vi "macro_BoolCmd_RecvMultiplexer.vi"() -> ()   [LabVIEW 2019, in "Trajectory_Library.lvlib"]
uses:
  VI/BoolCmd_Recv_Internal.vi
  VI/DigSeqLogic_Edge_On.vi
  VI/BoolCmd_ObtainQueue.vi
  Trajectory_Library.lvlib
panel:
  in  "Ready2":bool=TRUE
  out "Do Cancel":bool
  out "Do Command 2":bool
  out "Do Command 1":bool
  in  "Ready1":bool=TRUE
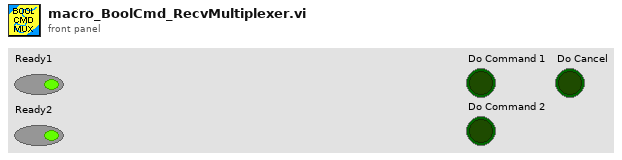
[diagram p1: front panel]
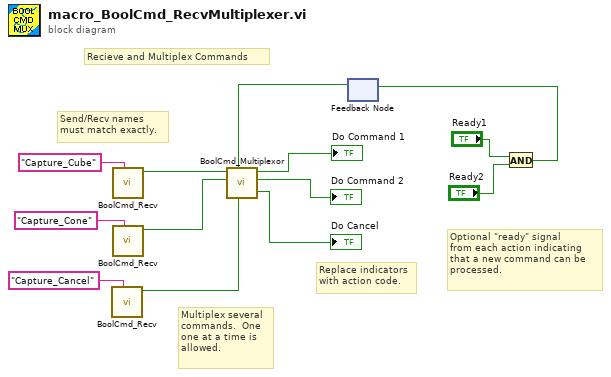
[diagram p0: block diagram]
diagram:
  # "Replace indicators\nwith action code."
  # "Optional \"ready\" signal\nfrom each action indicating\nthat a new command can be\nprocessed."
  # "Multiplex several\ncommands.  One\none at a time is \nallowed."
  # "Send/Recv names\nmust match exactly."
  # "Recieve and Multiplex Commands"
  n1 = call "BoolCmd_Recv.vi"("Command Name"="Capture_Cancel") -> ("New Request"=w8:bool)  [unwired: 9 in, 1 out]
  n2 = call "BoolCmd_Recv.vi"("Command Name"="Capture_Cube") -> ("New Request"=w10:bool)  [unwired: 9 in, 1 out]
  n3 = call "BoolCmd_Recv.vi"("Command Name"="Capture_Cone") -> ("New Request"=w9:bool)  [unwired: 9 in, 1 out]
  n4 = feedback #1() -> (w1:bool)  [unwired: 1 in]
  n5 = call "BoolCmd_Multiplexor.vi"("Command Cancel"=w8, "Ready"=w1, "Command 2"=w9, "Command 1"=w10) -> ("Do Command 2"=→"Do Command 2":bool, "Do Command 1"=→"Do Command 1":bool, "Do Cancel"=→"Do Cancel":bool)  [unwired: 3 in, 2 out]
  n6 = And(x="Ready1", y="Ready2") -> (x .and. y?=w2:bool)
  n7 = feedback-in #1(w2) -> ()
